vi "RadSensoren.vi"() -> ()   [LabVIEW 2016]
panel:
  out "vVL":dbl
  in  "vs":dbl
  out "vHL":sgl
  out "vHR":sgl
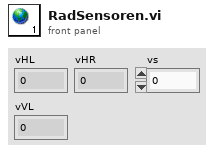
[diagram p1: front panel]
diagram:
